vi "Visable or not.vi"(4 "Result":T1) -> (1 "Boolean":bool)   [LabVIEW 2019]
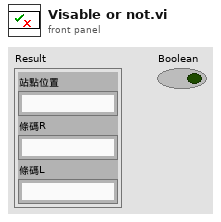
[diagram p1: front panel]
types:
  T1 = cluster{"站點位置":string, "條碼R":string, "條碼L":string}
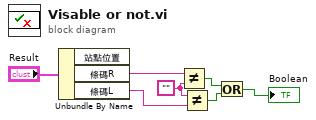
[diagram p0: block diagram]
diagram:
  w3 = ""
  n1 = Unbundle By Name("Result") -> ("條碼R"=w2:string, "條碼L"=w4:string)  [unwired: 1 out]
  n2 = Not Equal?(x=w2, y=w3) -> (x != y?=w5:bool)
  n3 = Not Equal?(x=w3, y=w4) -> (x != y?=w6:bool)
  n4 = Or(x=w5, y=w6) -> (x .or. y?=→"Boolean":bool)
